vi "CSM - Read Sections.vi"(7 "error in (no error)":errorcluster) -> (1 "error out":errorcluster, 3 "Sections":string[](array[string]))   [LabVIEW 2017, in "INI-Static-Variable-Support.lvlib"]
doc: "Reads all section names currently in memory.\n\n-- <b>Indicators</b> --\n- <b>Sections</b>: Array of section names."
uses:
  INI-Static-Variable-Support.lvlib
  _fgv-oper.ctl
  <userlib>/_NEVSTOP/Communicable State Machine(CSM)/_Support/ChangeFlag/ChangeFlag-Read.vi
  <userlib>/_NEVSTOP/Communicable State Machine(CSM)/_Support/ChangeFlag/ChangeFlagDB.vi
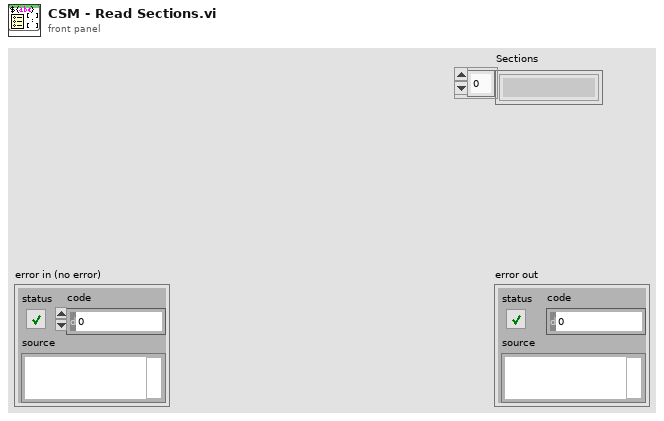
[diagram p1: front panel]
types:
  T1 = typedef "INI-Static-Variable-Support.lvlib/_fgv-oper.ctl" = enum16{"Read", "Write", "Sync", "Sessions", "List Keys", "Load", "List Files", "List Variables", "List Permanent Variables", "Mark Temp Variable as Permenent", "unload", "INIConfig(Memory)", "Reset", "Restore Variable Value"}
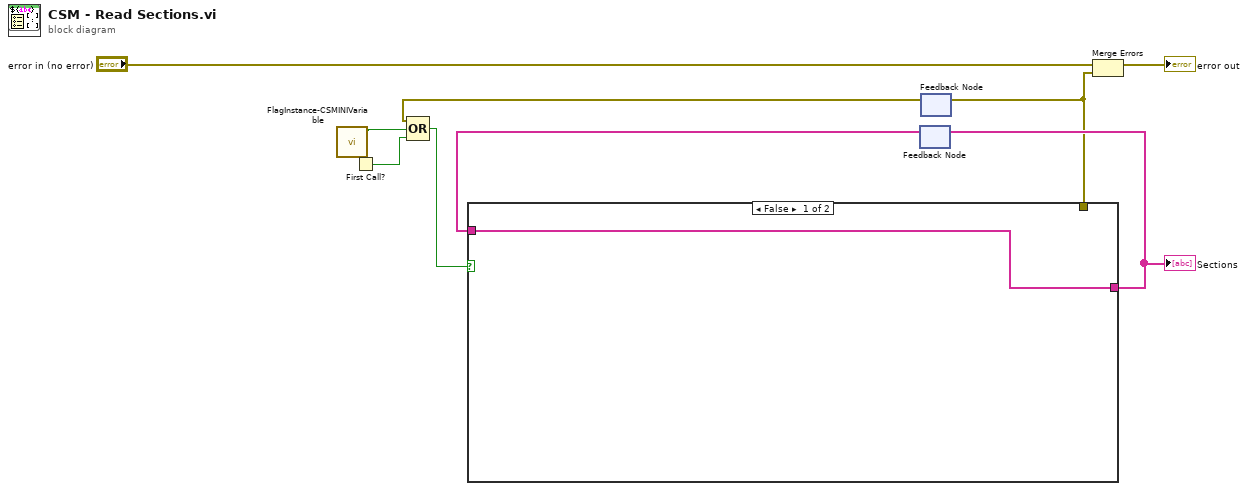
[diagram p0: block diagram]
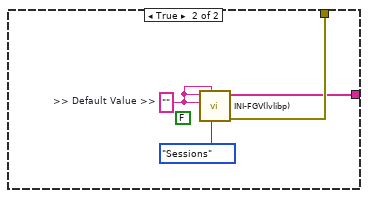
[diagram p2: hidden frame]
diagram:
  n1 = call "FlagInstance-CSMINIVariable.vi"() -> ("Changed"=w1:bool)  [unwired: 10 in, 1 out]
  n2 = First Call?() -> (First Call?: T/F=w2:bool)
  n3 = feedback #1() -> (w6:string[])  [unwired: 1 in]
  n4 = feedback #2() -> (w4:errorcluster)  [unwired: 1 in]
  n5 = Compound Arithmetic op=OR(w4, w1, w2) -> (w3:bool)
  n6 = case shown="False" w3 {
    tunnel: [_ w13] -> w5
    tunnel: [w10 w12] -> w7
    tunnel: w6 -> [w10 _]
    frame False {
    }
    frame True {
      w11 = ""  # >> Default Value >>
      (unwired) FALSE ("Raw String? (F)")
      n7 = call "INI-FGV(lvlibp).vi"("Enum"=_fgv-oper."Sessions", "Prefered Section"=w11, ">> Default Value >>"=w11, ">> Variable Name >>"=w11) -> ("error out"=w13:errorcluster, "Array"=w12:string[])  [unwired: 4 in, 2 out]
    }
  }
  "Sections" <- w7
  n8 = feedback-in #1(w7) -> ()
  n9 = feedback-in #2(w5) -> ()
  n10 = Merge Errors("error in (no error)", w5) -> (→"error out":errorcluster)
